vi "32Bit Two Complement.vi"(11 "Numeric in":u32) -> (3 "Numeric out":i32)   [LabVIEW 2014]
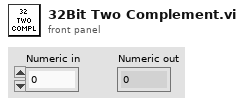
[diagram p1: front panel]
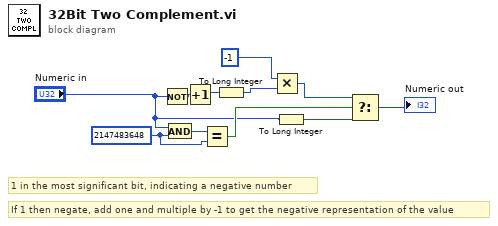
[diagram p0: block diagram]
diagram:
  w6 = u32 2147483648 ("y")
  # "If 1 then negate, add one and multiple by -1 to get the negative representation of the value"
  # "1 in the most significant bit, indicating a negative number"
  n1 = Not(x="Numeric in") -> (.not. x?=w9:u32)
  n2 = And(x="Numeric in", y=w6) -> (x .and. y?=w5:u32)
  n3 = Increment(x=w9) -> (x+1=w2:u32)
  n4 = Equal?(x=w5, y=w6) -> (x = y?=w7:bool)
  n5 = To Long Integer(number=w2) -> (32bit integer=w1:i32)
  n6 = Multiply(x=-1, y=w1) -> (x*y=w11:i32)
  n7 = To Long Integer(number="Numeric in") -> (32bit integer=w3:i32)
  n8 = Select(t=w11, s=w7, f=w3) -> (s? t:f=→"Numeric out":i32)
